vi "Get Write Decimation.vi"(8 "error in (no error)":errorcluster, 11 "Custom Device reference in":refnum<k24>) -> (0 "error out":errorcluster, 2 "Write Decimation":u32, 3 "Custom Device reference out":refnum<k24>)   [LabVIEW 2019, in "J1939 System Definition API Support.lvlib"]
uses:
  J1939 System Definition API Support.lvlib
  Shared/SubVIs/Constants.vi
  Shared/J1939 Addon Shared.lvlib
  <vilib>/NI VeriStand/Custom Device API/Custom Device API.lvlib
  <vilib>/NI VeriStand/Custom Device API/Get Item Property (Variant).vi
  Shared/Types/XNET Settings.ctl
  NationalInstruments.VeriStand.SystemDefinitionAPI
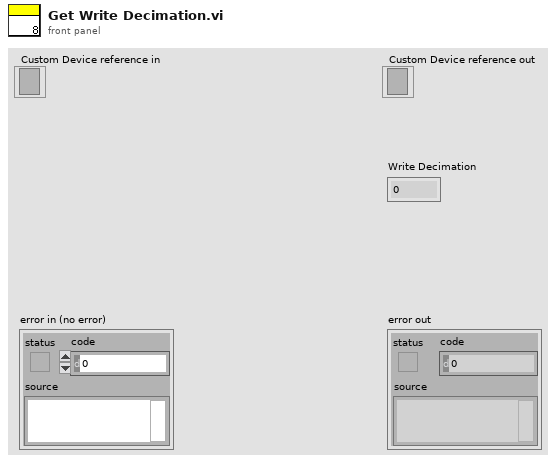
[diagram p1: front panel]
types:
  T1 = typedef "J1939 Addon Shared.lvlib/XNET Settings.ctl" = cluster{"Database":refnum<k21>, "Cluster":refnum<k21>, "Port":string, "Baud rate [Bd]":u32, "Termination":u32, "Incoming Decimation":u32, "Outgoing Decimation":u32}
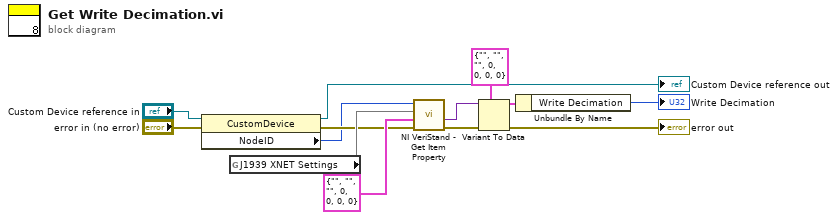
[diagram p0: block diagram]
diagram:
  n1 = property class="CustomDevice"(reference="Custom Device reference in", error in="error in (no error)") -> (reference out=→"Custom Device reference out":refnum<k24>, error out=w5:errorcluster, "NodeID"=w1:u64)
  n2 = global read "Constants.vi" "J1939 XNET Settings"() -> (w10)
  n3 = call-poly <vilib>:"NI VeriStand - Get Item Property.vi"("error in (no error)"=w5, "Default Value"=T1 {"Database"="", "Cluster"="", "Port"="", "Baud rate [Bd]"=0, "Termination"=0, "Incoming Decimation"=0, "Outgoing Decimation"=0} ("J1939 XNET Settings"), "Property Name"=w10, "Item Ref in"=w1) -> ("error out"=w9:errorcluster, "Value"=w8:variant)  [unwired: 4 in, 2 out]
  n4 = Variant To Data(error in=w9, type=T1 {"Database"="", "Cluster"="", "Port"="", "Baud rate [Bd]"=0, "Termination"=0, "Incoming Decimation"=0, "Outgoing Decimation"=0} ("J1939 XNET Settings"), Variant=w8) -> (data=w3:T1, error out=→"error out":errorcluster)
  n5 = Unbundle By Name(w3) -> ("Write Decimation"=→"Write Decimation":u32)
